vi "Less Than.vi"(1 "comparable b":string, 2 "comparable a":string) -> (0 "less?":bool)   [LabVIEW 2020, in "AoC 2022.lvlib"]
doc: "Returns whether <b>comparable a</b> is less than <b>comparable b</b>."
uses:
  AoC 2022.lvlib
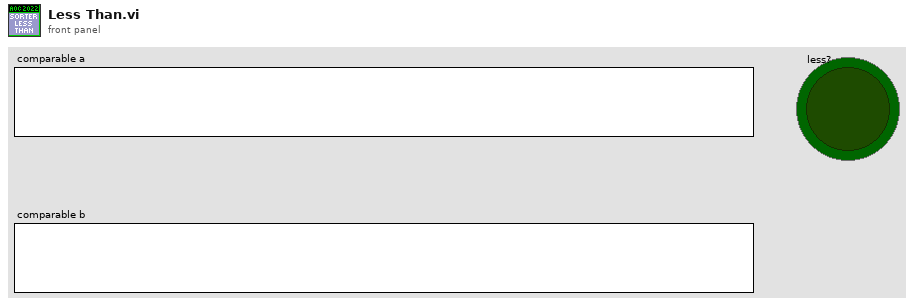
[diagram p1: front panel]
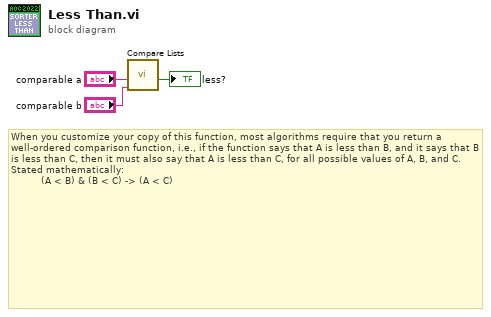
[diagram p0: block diagram]
diagram:
  # "When you customize your copy of this function, most algorithms require that you return a well-ordered comparison function, i.e., if the function says that A is less than B, and it says that B is less than C, then it must also say that A is less than C, for all possible values of A, B, and C. Stated mathematically:\n          (A < B) & (B < C) -> (A < C)"
  n1 = call "Compare Lists.vi"("Right List"="comparable b", "Left List"="comparable a") -> ("In Right Order ?"=→"less?":bool)  [unwired: 2 in, 3 out]
